vi "IDdatadirectory.vi"(8 "Read path automatically from:":path, 9 "Directory":string, 10 "Save path":path, 11 "Manual or automatic":bool) -> (3 "Outputpath":path)   [LabVIEW 2009]
panel:
  out "String 3":string
  out "String 2":string
  out "String":string
  out "Outputpath 3":path
  out "Outputpath 2":path
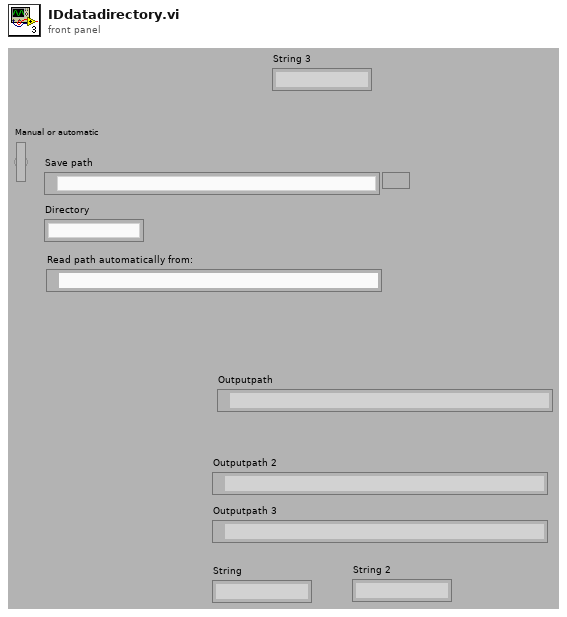
[diagram p1: front panel]
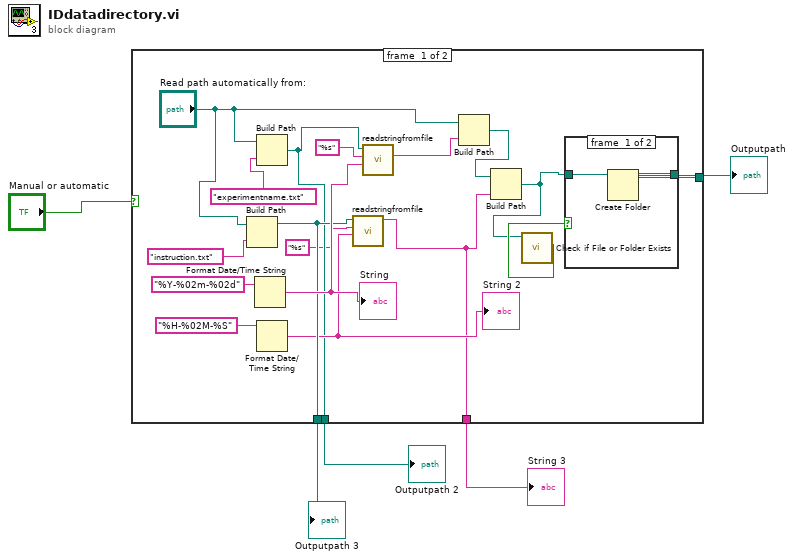
[diagram p0: block diagram]
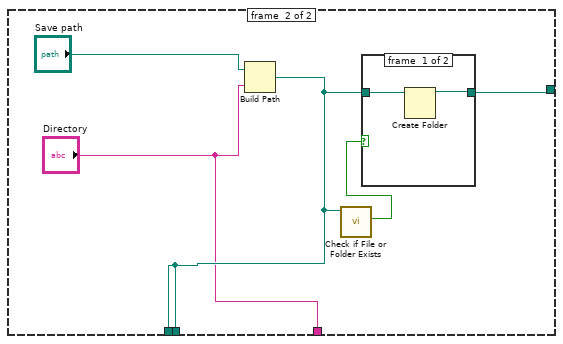
[diagram p3: hidden frame]
diagram:
  n1 = case shown="False" "Manual or automatic" {
    tunnel: [w8 w27] -> w4
    tunnel: [w11 w29] -> w3
    tunnel: [w13 w29] -> w2
    tunnel: [w7 "Directory"] -> w1
    frame #0 {
      n2 = Build Path(base path="Read path automatically from:", name or relative path="instruction.txt") -> (appended path=w13:path)
      n3 = Format Date/Time String(time format string (%c)="%Y-%02m-%02d") -> (date/time string=w19:string)  [unwired: 2 in]
      "String" <- w19
      n4 = Build Path(base path="Read path automatically from:", name or relative path="experimentname.txt") -> (appended path=w11:path)
      n5 = Format Date/Time String(time format string (%c)="%H-%02M-%S") -> (date/time string=w12:string)  [unwired: 2 in]
      "String 2" <- w12
      n6 = call "readstringfromfile.vi"("default value"=w12, "Format string"="%s" ("format string"), "Filename to read from:"=w13) -> ("output string"=w7:string)  [unwired: 8 in]
      n7 = call "readstringfromfile.vi"("default value"=w19, "Format string"="%s" ("format string"), "Filename to read from:"=w11) -> ("output string"=w16:string)  [unwired: 8 in]
      n8 = Build Path(base path="Read path automatically from:", name or relative path=w16) -> (appended path=w14:path)
      n9 = Build Path(base path=w14, name or relative path=w7) -> (appended path=w9:path)
      n10 = call <vilib>:"Check if File or Folder Exists.vi"("path"=w9) -> ("file or folder exists?"=w10:bool)  [unwired: 8 in, 2 out]
      n11 = case shown="True" w10 {
        tunnel: w9 -> [w24 w25]
        tunnel: [w23 w25] -> w8
        frame #0 {
          n12 = Create Folder(path (use dialog)=w24) -> (created path=w23:path)  [unwired: 2 in, 2 out]
        }
        frame #1 {
        }
      }
    }
    frame #1 {
      n13 = Build Path(base path="Save path", name or relative path="Directory") -> (appended path=w29:path)
      n14 = call <vilib>:"Check if File or Folder Exists.vi"("path"=w29) -> ("file or folder exists?"=w28:bool)  [unwired: 8 in, 2 out]
      n15 = case shown="False" w28 {
        tunnel: w29 -> [w31 w33]
        tunnel: [w32 w33] -> w27
        frame #0 {
          n16 = Create Folder(path (use dialog)=w31) -> (created path=w32:path)  [unwired: 2 in, 2 out]
        }
        frame #1 {
        }
      }
    }
  }
  "Outputpath" <- w4
  "Outputpath 2" <- w3
  "Outputpath 3" <- w2
  "String 3" <- w1
